vi "gfitsio-read-record.vi"(7 "nrec":i32, 8 "error in (no error)":errorcluster, 11 "gfits refnum":T1) -> (0 "error out":errorcluster, 2 "card":string, 3 "dup gfits refnum":T1)   [LabVIEW 2023, in "gfitsio.lvlib"]
doc: "Return the nth header record in the HDU; the first keyword in the header is 1."
uses:
  gfitsio.lvlib
  gfitsio.dll
  gfitsio-refnum.ctl
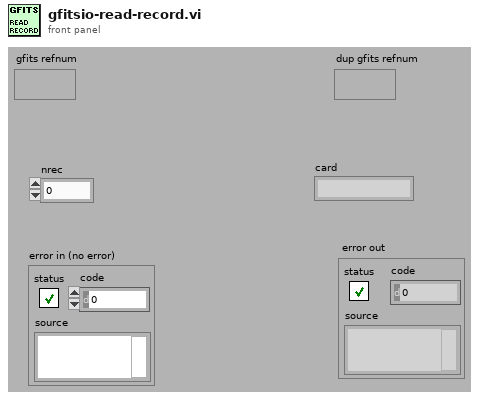
[diagram p1: front panel]
types:
  T1 = typedef "gfitsio.lvlib/gfitsio-refnum.ctl" = refnum<k1>
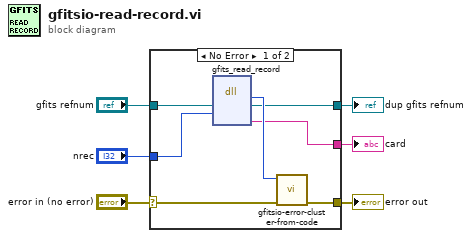
[diagram p0: block diagram]
diagram:
  n1 = case shown="No Error" "error in (no error)" {
    selector: "error in (no error)" -> [w12 w15]
    tunnel: [w11 w15] -> w6
    tunnel: "gfits refnum" -> [w9 w14]
    tunnel: [w10 w14] -> w4
    tunnel: [w8 _] -> w2
    tunnel: "nrec" -> [w7 _]
    frame No Error {
      n2 = dll-call lib="gfitsio.dll" fn="gfits_read_record"("refnum"=w9, "nrec"=w7) -> (w13:i32, "refnum"=w10:T1, "card"=w8:string)  [unwired: 4 in, 3 out]
      n3 = call "gfitsio-error-cluster-from-code.vi"("error in (no error)"=w12, "error code"=w13) -> ("error out"=w11:errorcluster)  [unwired: 9 out]
    }
    frame Error {
    }
  }
  "error out" <- w6
  "dup gfits refnum" <- w4
  "card" <- w2
